vi "saveData.vi"   [LabVIEW 2017]
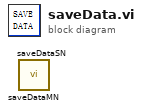
[diagram p0: block diagram]
diagram:
  n1 = call "saveDataMN.vi"() -> ()  [unwired: 11 in, 1 out]
  n2 = call "saveDataSN.vi"() -> ()  [unwired: 11 in, 1 out]
